vi "Initialize Private Data.vi"(10 "BG Color":u32(colorbox)) -> (3 "Ex Event Actor out":refnum<class "Ex Event Actor.lvclass">)   [LabVIEW 2021, in "Ex Event Actor.lvlib" / "Ex Event Actor.lvclass"]
uses:
  Ex Event Actor.lvclass
  Ex Event Actor.lvclass/Ex Event Actor.ctl
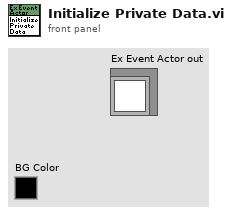
[diagram p1: front panel]
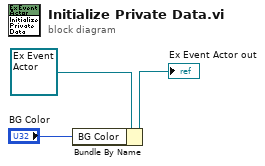
[diagram p0: block diagram]
diagram:
  n1 = Bundle By Name(cluster=refnum<class "Ex Event Actor.lvclass"> refnum ("Dev Panel in"), "BG Color"="BG Color") -> (→"Ex Event Actor out":refnum<class "Ex Event Actor.lvclass">)
